vi "test harness_FXP_Linear_control_law.vi"(8 "error in (no error)":errorcluster, 11 "TestCase in":refnum<class "FXP_observer_TestCase.lvclass">) -> (0 "error out":errorcluster, 3 "TestCase out":refnum<class "FXP_observer_TestCase.lvclass">)   [LabVIEW 2017, in "FXP_observer_TestCase.lvclass"]
uses:
  FXP_observer_TestCase.lvclass
  <vilib>/rvi/DesktopExecutionNode/DesktopExecutionNode.xnode
  <vilib>/rvi/DesktopExecutionNode/Execution/niFpgaDEN_Execute.vi
  fpga_VIs/fixed-point/typeDefs/x_vec_type.ctl
panel:
  in  "xk_12":T1=[0.0, 0.0, 0.0, 0.0, 0.0, 0.0, 0.0, 0.0, 0.0, 0.0, 0.0, 0.0, 0.0, 0.0, 0.0, 0.0, 0.0, 0.0, 0.0, 0.0, 0.0, 0.0, 0.0, 0.0, 0.0]
  out "xerr(expected)":fxp<+/-,64,11>[](array[numeric])
  out "x*y":fxp<+/-,64,10>[](array[numeric])
  out "xerr":fxp<+/-,32,8>[](array[numeric])
  in  "yd_est":fxp<+/-,32,5>
  out "error (xerr)":errorcluster
  out "delta uk (expected)":dbl
  out "del u(k)":fxp<+/-,64,15>
  out "error (delta uk)":errorcluster
  in  "du_umax":fxp<+/-,18,5>=10.0
  in  "ControlParams_distEst":T2={"umax"=0.0, "NS"=22, "ref_f_VEC"=[0.0, 0.0], "Nu11_22"=[0.0, 0.0], "u0"=[0.0, 0.0]}
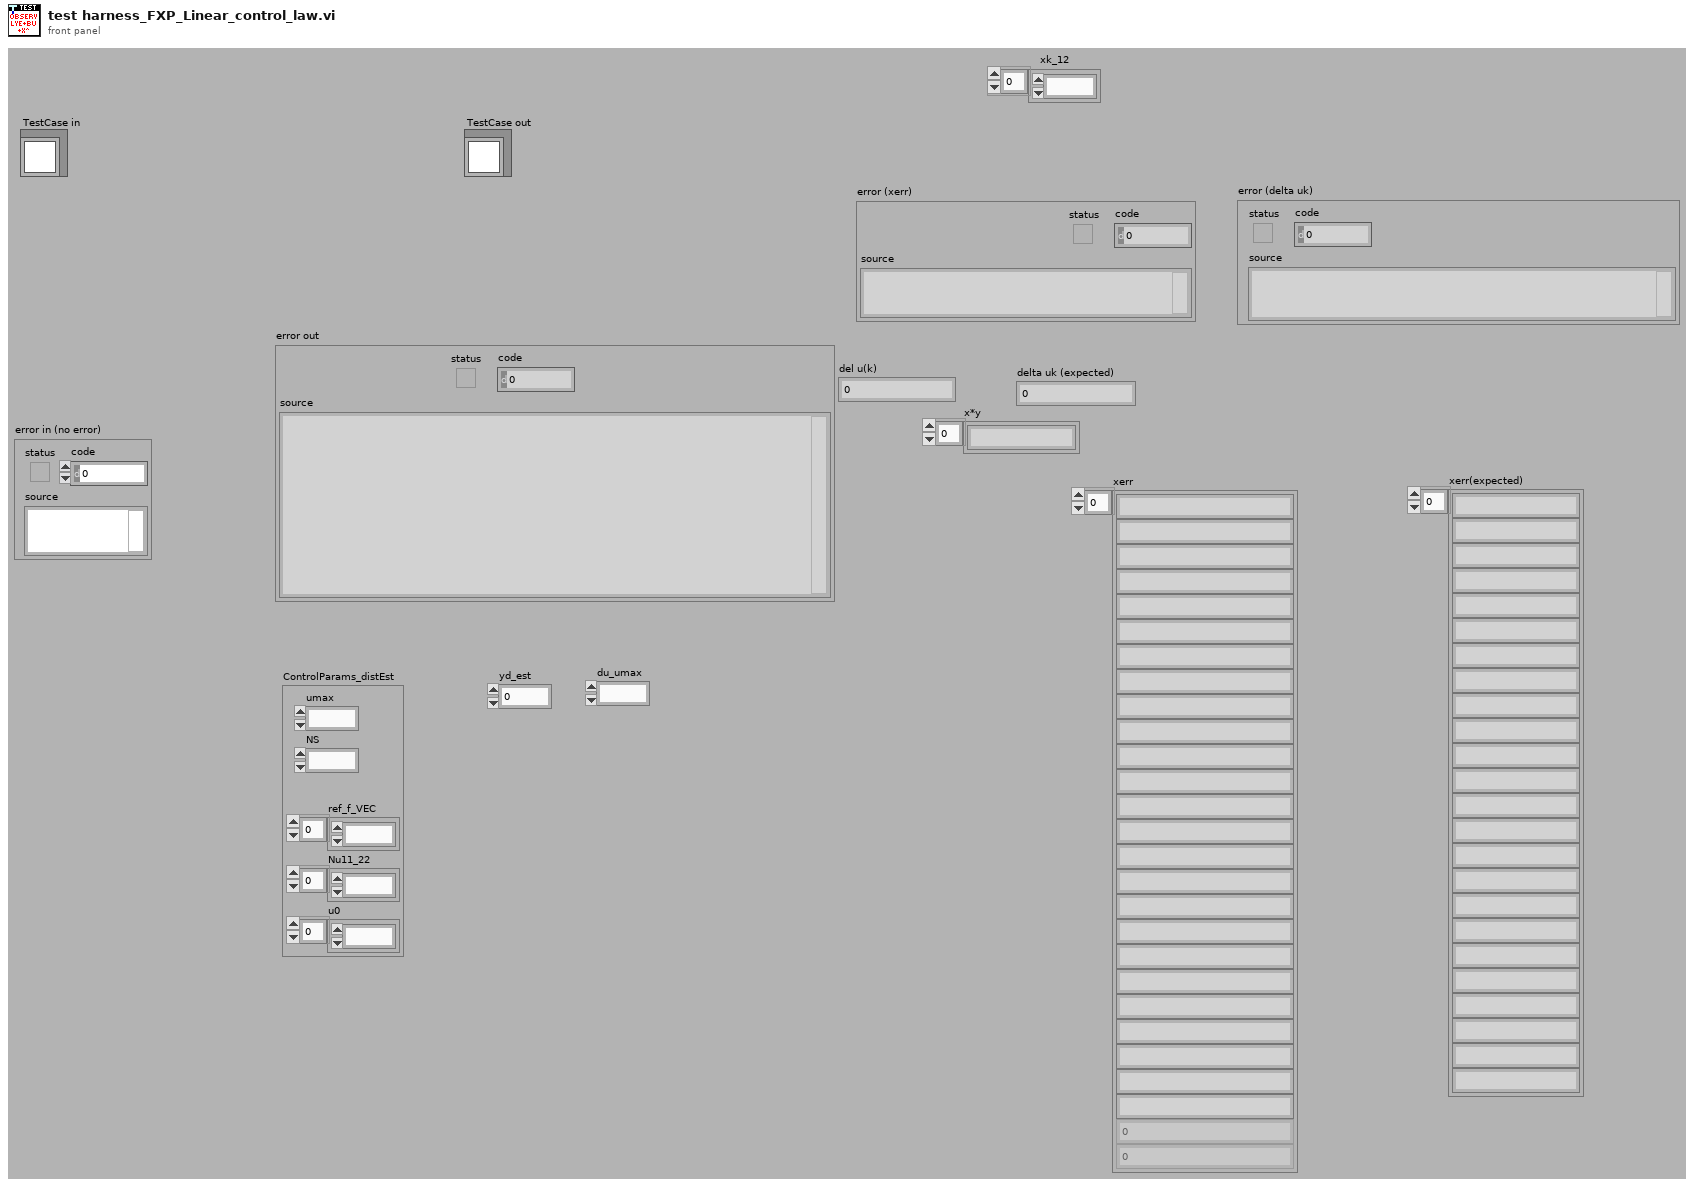
[diagram p1: front panel]
types:
  T1 = typedef "x_vec_type.ctl" = fxp<+/-,32,6>[]
  T2 = cluster{"umax":fxp<+/-,18,5>, "NS":u8, "ref_f_VEC":fxp<+/-,32,5>[], "Nu11_22":fxp<+/-,32,5>[], "u0":fxp<+/-,32,5>[]}
  T3 = typedef "UT_matrix_data.ctl" = cluster{"Bz":T4[], "Ldist":T5[], "Kz":T6[], "Nx":T7[], "Ax_col":T8[], "X_vec":T9[], "Cz":T10[]}
  T4 = typedef "Bz_vec_scalar.ctl" = fxp<+/-,32,3>
  T5 = typedef "Lz_vec_scalar.ctl" = fxp<+/-,32,3>
  T6 = typedef "Kz_vec_scalar.ctl" = fxp<+/-,32,10>
  T7 = typedef "Nx_vec_scalar.ctl" = fxp<+/-,32,2>
  T8 = typedef "Az_vec_scalar.ctl" = fxp<+/-,32,7>
  T9 = typedef "x_vec_scalar.ctl" = fxp<+/-,32,6>
  T10 = typedef "Cz_vec_scalar.ctl" = fxp<+/-,32,4>
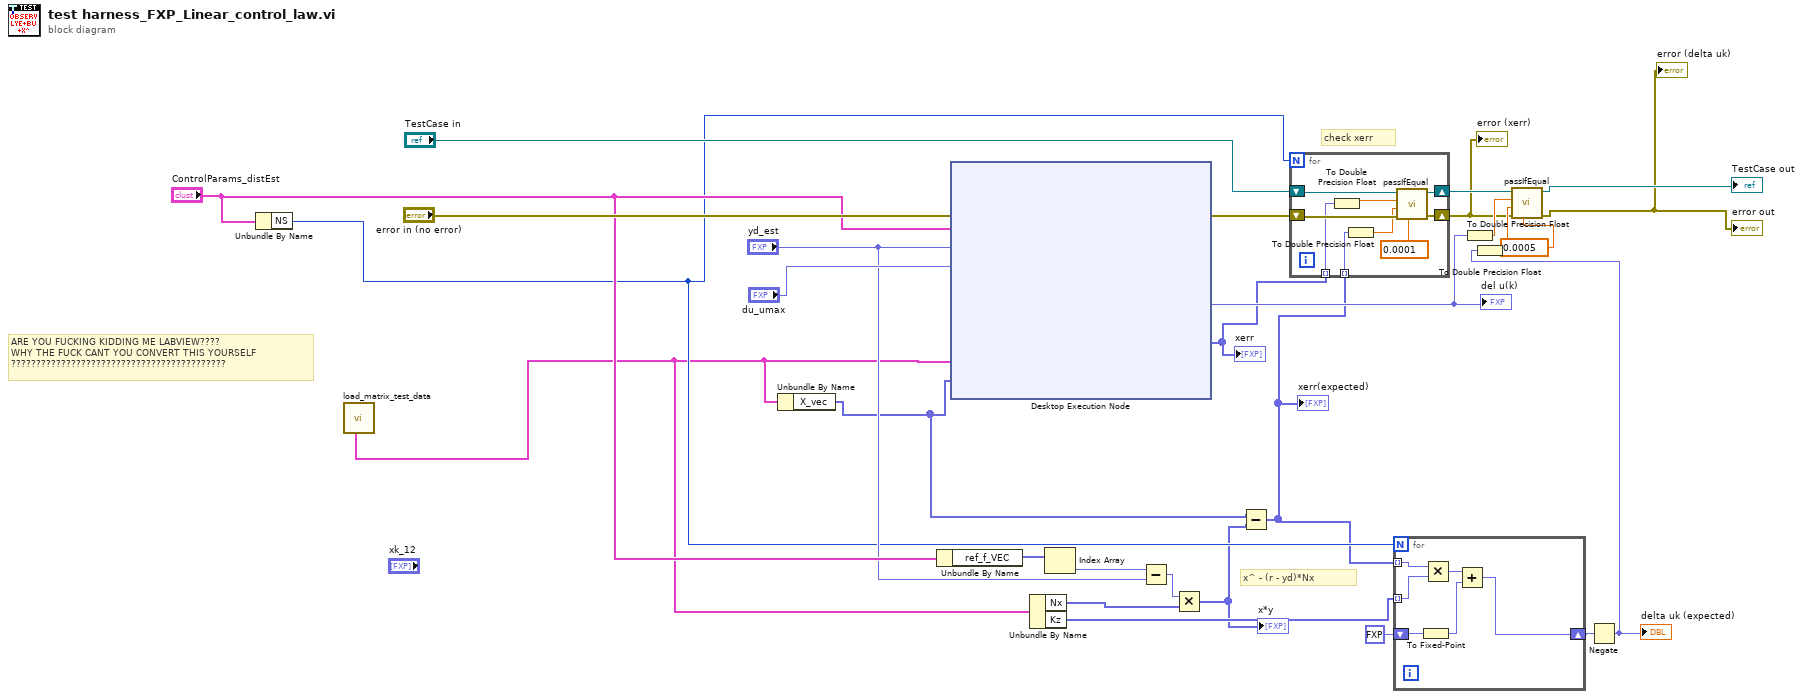
[diagram p0: block diagram]
diagram:
  # "x^ - (r - yd)*Nx"
  # "check xerr"
  # "ARE YOU FUCKING KIDDING ME LABVIEW????\nWHY THE FUCK CANT YOU CONVERT THIS YOURSELF\n???????????????????????????????????????????"
  n1 = Unbundle By Name("ControlParams_distEst") -> ("NS"=w7:u8)
  n2 = call "load_matrix_test_data.vi"() -> ("output cluster"=w2:T3)  [unwired: 5 in, 6 out]
  n3 = Unbundle By Name(w2) -> ("X_vec"=w1:T9[])
  n4 = Unbundle By Name("ControlParams_distEst") -> ("ref_f_VEC"=w25:fxp<+/-,32,5>[])
  n5 = xnode "Desktop Execution Node"("Error In"="error in (no error)", "ControlParams_distEst"="ControlParams_distEst", "yd_est"="yd_est", "du_umax"="du_umax", "Matrix Data"=w2, "xk_12"=w1) -> ("Error Out"=w17:errorcluster, "del u(k)"=w11:fxp<+/-,64,15>, "xerr"=w5:fxp<+/-,32,6>[])  [unwired: 2 out]
  "del u(k)" <- w11
  "xerr" <- w5
  n6 = Unbundle By Name(w2) -> ("Nx"=w26:T7[], "Kz"=w23:T6[])
  n7 = Index Array(array=w25) -> (element=w24:fxp<+/-,32,5>)  [unwired: 1 in]
  n8 = Subtract(x=w24, y="yd_est") -> (x-y=w27:fxp<+/-,32,5>)
  n9 = Multiply(x=w27, y=w26) -> (x*y=w3:fxp<+/-,64,10>[])
  "x*y" <- w3
  n10 = Subtract(x=w1, y=w3) -> (x-y=w4:T9[])
  "xerr(expected)" <- w4
  n11 = for {
    N: w7 -> [_]
    shift-right: [w37] -> w15
    shift-left: "TestCase in" -> [w34]
    shift-right: [w36] -> w8
    shift-left: w17 -> [w35]
    tunnel: w4 -> [w31] mode=indexing
    tunnel: w5 -> [w30] mode=indexing
    n12 = To Double Precision Float(number=w30) -> (double precision float=w32:dbl)
    n13 = To Double Precision Float(number=w31) -> (double precision float=w33:dbl)
    n14 = call-dynamic "passIfEqual.vi"("delta (optional)"=0.0001 ("del u_x"), "error in (no error)"=w35, "y"=w33, "x"=w32, "TestCase in"=w34) -> ("error out"=w36:errorcluster, "TestCase out"=w37:refnum<class "FXP_observer_TestCase.lvclass">)  [unwired: 5 in]
  }
  "error (xerr)" <- w8
  n15 = for {
    N: w7 -> [_]
    tunnel: w4 -> [w43] mode=indexing
    tunnel: w23 -> [w42] mode=indexing
    shift-right: [w40] -> w21
    shift-left: fxp<+,32,5> 0.0 -> [w39]
    n16 = To Fixed-Point(number=w39) -> (fixed-point=w38:fxp<+/-,64,15>)  [unwired: 1 in]
    n17 = Multiply(x=w43, y=w42) -> (x*y=w41:fxp<+/-,64,16>)
    n18 = Add(x=w41, y=w38) -> (x+y=w40:fxp<+/-,64,16>)
  }
  n19 = To Double Precision Float(number=w11) -> (double precision float=w14:dbl)
  n20 = Negate(x=w21) -> (-x=w12:fxp<+/-,64,17>)
  "delta uk (expected)" <- w12
  n21 = To Double Precision Float(number=w12) -> (double precision float=w13:dbl)
  n22 = call-dynamic "passIfEqual.vi"("delta (optional)"=0.0005 ("del u_x"), "error in (no error)"=w8, "y"=w13, "x"=w14, "TestCase in"=w15) -> ("error out"=→"error out" →"error (delta uk)":errorcluster, "TestCase out"=→"TestCase out":refnum<class "FXP_observer_TestCase.lvclass">)  [unwired: 5 in]
